vi "בדיקת צריכת זרם של סליל הפיקוד 4.vi"(7 "resultUserPrompt":bool, 8 "error":errorcluster, 11 "Path for Log":path) -> (0 "error out":errorcluster, 2 "צריכת זרם בסליל בטווח כן/לא":bool, 3 "צריכת זרם בסליל":dbl format="%.4f")   [LabVIEW 2015]
uses:
  <vilib>/DAQmx/write.llb/DAQmx Write (Digital Bool 1Line 1Point).vi
  <vilib>/DAQmx/create/channels.llb/DAQmx Create Channel (DO-Digital Output).vi
  <vilib>/DAQmx/miscellaneous.llb/DAQmx Fill In Error Info.vi
panel:
  # "Right-Click to\nexplain error"
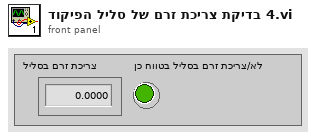
[diagram p1: front panel]
types:
  T1 = enum32{"Invalid", "Standard", "Closed", "Hidden", "Minimized", "Maximized"}
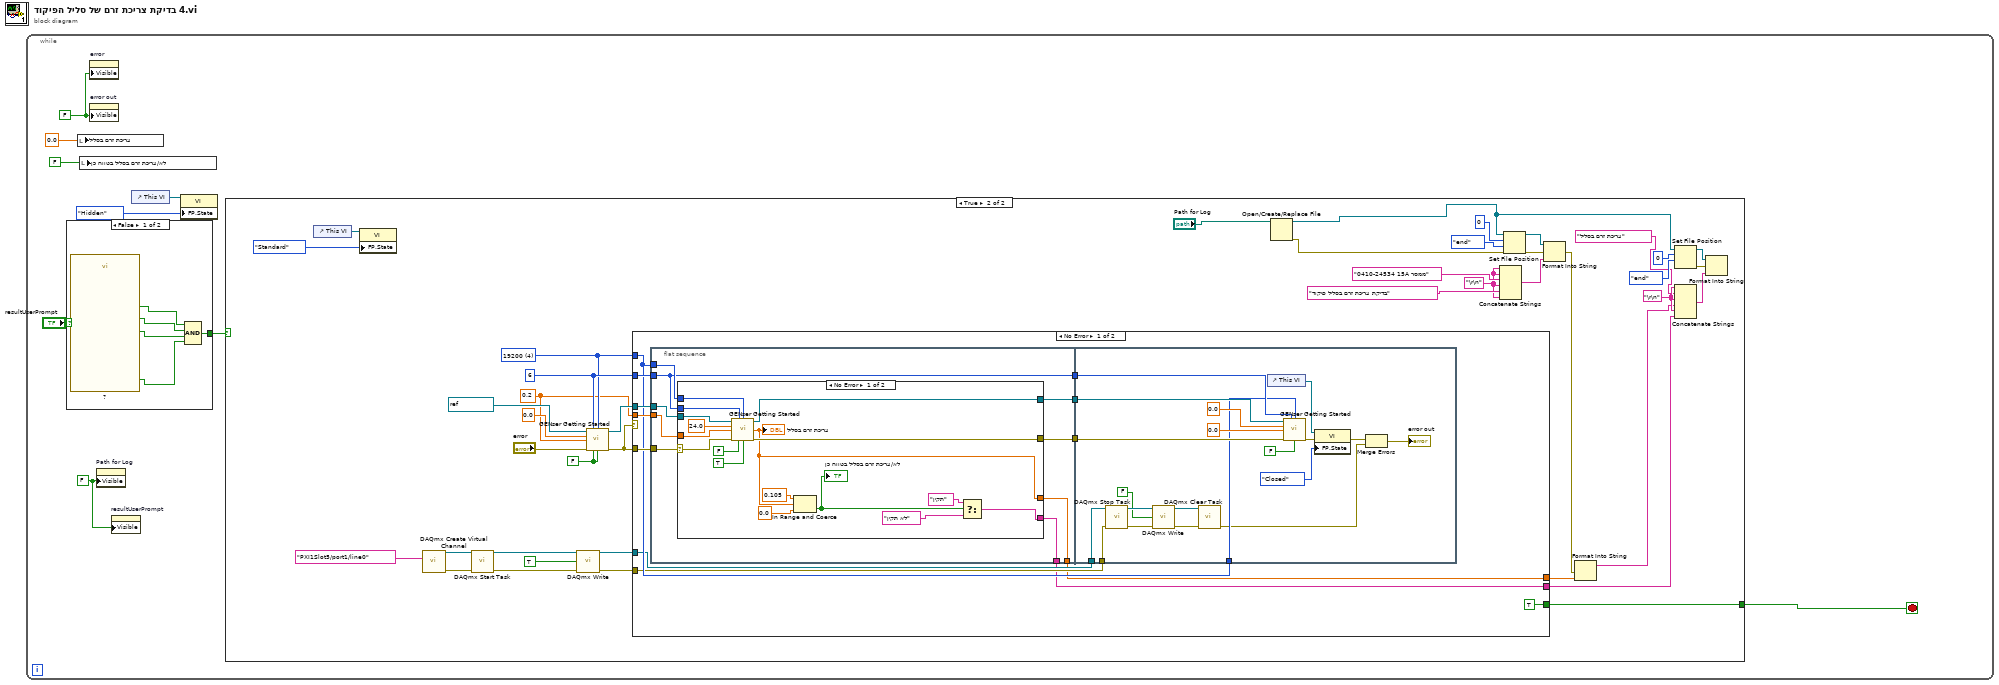
[diagram p0: block diagram]
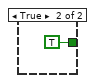
[diagram p2: hidden frame]
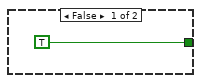
[diagram p3: hidden frame]
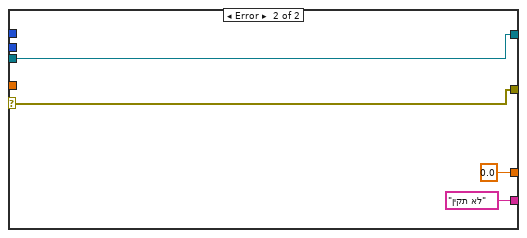
[diagram p4: hidden frame]
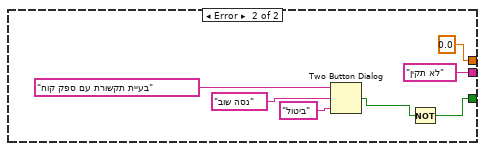
[diagram p5: hidden frame]
diagram:
  n1 = while {
    stop <- w1 stop-if-true
    w2 = FALSE ("Visible")
    w6 = FALSE ("Visible")
    n2 = case shown="False" "resultUserPrompt" {
      tunnel: [w14 TRUE] -> w9
      frame False {
        n3 = call "?"() -> ("הדקי הרב מודד"=w10:bool, "(מגע שלילי (מעטפת"=w11:bool, "A מגע חיובי"=w12:bool, "OK"=w13:bool)  [unwired: 15 in, 1 out]
        n4 = Compound Arithmetic op=AND(w13, w12, w11, w10) -> (w14:bool)
      }
      frame True {
      }
    }
    n5 = local write "צריכת זרם בסליל"(0.0 ("Output Current")) -> ()
    n6 = local write "צריכת זרם בסליל בטווח כן/לא"(FALSE ("In Range?")) -> ()
    n7 = property on="error" class="Clust (strict)"("Visible"=w6) -> ()  [unwired: 2 in, 2 out]
    n8 = property on="error out" class="Clust (strict)"("Visible"=w6) -> ()  [unwired: 2 in, 2 out]
    n9 = property on="Path for Log" class="Path"("Visible"=w2) -> ()  [unwired: 2 in, 2 out]
    n10 = property on="resultUserPrompt" class="Bool (strict)"("Visible"=w2) -> ()  [unwired: 2 in, 2 out]
    n11 = control-ref of="This VI"() -> (w5:refnum<vi>)
    n12 = property class="VI"(reference=w5, "FP.State"=T1."Hidden" ("Front Panel Window:State")) -> ()  [unwired: 1 in, 2 out]
    n13 = case shown="True" w9 {
      tunnel: [TRUE ("T button?") w50] -> w1
      frame False {
      }
      frame True {
        w23 = "\r\n"
        w32 = "\r\n"
        w49 = FALSE ("Output On (T)")
        w54 = u16 4 items=["1200", "2400", "4800", "9600", "19200"] ("BAUD")
        w55 = i16 6 ("GEN Addr")
        w51 = 0.2 ("Current Limit")
        n14 = control-ref of="This VI"() -> (w48:refnum<vi>)
        n15 = property class="VI"(reference=w48, "FP.State"=T1."Standard" ("Front Panel Window:State")) -> ()  [unwired: 1 in, 2 out]
        n16 = call-poly <vilib>:"DAQmx Create Virtual Channel.vi"("lines"=tag "PXI1Slot5/port1/line0") -> ("task out"=w45:refnum<k21>, "error out"=w46:errorcluster)  [unwired: 13 in]
        n17 = call <vilib>:"DAQmx Start Task.vi"("task/channels in"=w45, "error in"=w46) -> ("task out"=w43:refnum<k21>, "error out"=w42:errorcluster)  [unwired: 12 in]
        n18 = call-poly <vilib>:"DAQmx Write.vi"("task/channels in"=w43, "data"=TRUE, "error in"=w42) -> ("task out"=w40:refnum<k21>, "error out"=w39:errorcluster)  [unwired: 10 in, 1 out]
        n19 = call "GENser Getting Started.vi"("VISA"=refnum<visa-resource-name> "COM6", "GEN Addr"=w55, "BAUD"=w54, "Voltage Limit"=0.0, "Current Limit"=w51, "error"="error", "Reset (T)"=w49, "Output On (T)"=w49) -> ("VISA out"=w56:refnum<visa-resource-name>, "error out"=w57:errorcluster)  [unwired: 4 in, 2 out]
        n20 = case shown="No Error" w57 {
          tunnel: w57 -> [w66 _]
          tunnel: w56 -> [w68 _]
          tunnel: w55 -> [w69 _]
          tunnel: w54 -> [w63 _]
          tunnel: w51 -> [w67 _]
          tunnel: [TRUE w122] -> w50
          tunnel: w40 -> [w62 _]
          tunnel: w39 -> [w61 _]
          tunnel: [w60 0.0 ("Output Current")] -> w29
          tunnel: [w59 "לא תקין"] -> w21
          frame No Error {
            n21 = flat-sequence {
              tunnel: [w80] -> w70
              tunnel: w63 -> [w79]
              tunnel: w69 -> [w75]
              tunnel: w68 -> [w78]
              tunnel: w67 -> [w77]
              tunnel: w66 -> [w74]
              tunnel: [w76] -> w65
              tunnel: [w75] -> w64
              tunnel: [w73] -> w60
              tunnel: [w72] -> w59
              tunnel: w70 -> [w118]
              tunnel: w65 -> [w117]
              tunnel: w64 -> [w116]
              tunnel: w63 -> [w115]
              tunnel: w62 -> [w103]
              tunnel: w61 -> [w102]
              frame #0 {
                n22 = case shown="No Error" w74 {
                  selector: w74 -> [w86 w100]
                  tunnel: [w92 w100] -> w80
                  tunnel: w79 -> [w91 _]
                  tunnel: w75 -> [w90 _]
                  tunnel: w78 -> [w89 w101]
                  tunnel: w77 -> [w88 _]
                  tunnel: [w87 w101] -> w76
                  tunnel: [w85 0.0 ("Output Current")] -> w73
                  tunnel: [w81 "לא תקין"] -> w72
                  frame No Error {
                    n23 = call "GENser Getting Started.vi"("VISA"=w89, "GEN Addr"=w90, "BAUD"=w91, "Voltage Limit"=24.0, "Current Limit"=w88, "error"=w86, "Reset (T)"=FALSE, "Output On (T)"=TRUE) -> ("VISA out"=w87:refnum<visa-resource-name>, "Output Current"=w85:dbl, "error out"=w92:errorcluster)  [unwired: 4 in, 1 out]
                    "צריכת זרם בסליל" <- w85
                    n24 = In Range and Coerce(upper limit=0.105, x=w85, lower limit=0.0) -> (In Range?=w82:bool)  [unwired: 1 out]
                    "צריכת זרם בסליל בטווח כן/לא" <- w82
                    n25 = Select(t="תקין", s=w82, f="לא תקין") -> (s? t:f=w81:string)
                  }
                  frame Error {
                  }
                }
              }
              frame #1 {
                n26 = call <vilib>:"DAQmx Stop Task.vi"("task/channels in"=w103, "error in"=w102) -> ("task out"=w111:refnum<k21>, "error out"=w110:errorcluster)  [unwired: 12 in]
                n27 = call-poly <vilib>:"DAQmx Write.vi"("task/channels in"=w111, "data"=FALSE, "error in"=w110) -> ("task out"=w109:refnum<k21>, "error out"=w108:errorcluster)  [unwired: 10 in, 1 out]
                n28 = call <vilib>:"DAQmx Clear Task.vi"("task in"=w109, "error in"=w108) -> ("error out"=w105:errorcluster)  [unwired: 13 in]
                n29 = control-ref of="This VI"() -> (w114:refnum<vi>)
                n30 = call "GENser Getting Started.vi"("VISA"=w117, "GEN Addr"=w116, "BAUD"=w115, "Voltage Limit"=0.0, "Current Limit"=0.0, "error"=w118, "Output On (T)"=FALSE) -> ("error out"=w112:errorcluster)  [unwired: 5 in, 3 out]
                n31 = property class="VI"(reference=w114, error in=w112, "FP.State"=T1."Closed" ("Front Panel Window:State")) -> (error out=w106:errorcluster)  [unwired: 1 out]
                n32 = Merge Errors(w106, w105) -> (→"error out":errorcluster)
              }
            }
          }
          frame Error {
            n33 = Two Button Dialog(message="בעיית תקשורת עם ספק קוח", 1:"ביטול" ("F button name (\"Cancel\")"), 2:"נסה שוב" ("T button name (\"OK\")")) -> (T button?=w123:bool)
            n34 = Not(x=w123) -> (.not. x?=w122:bool)
          }
        }
        n35 = Open/Create/Replace File(file path (use dialog)="Path for Log") -> (refnum out=w17:refnum<file>, error out=w18:errorcluster)  [unwired: 5 in, 1 out]
        n36 = Concatenate Strings(w32, w32, "0410-24534 15A ממסר", w32, "בדיקת צריכת זרם בסליל פיקוד", w32) -> (w36:string)
        n37 = Set File Position(offset (in bytes) (0)=i64 0, refnum=w17, from (0:start)=enum16{"start", "end", "current"}."end", error in=w18) -> (refnum out=w33:refnum<file>, error out=w31:errorcluster)
        n38 = Format Into String(initial string=w33, error in=w31, w36) -> (error out=w30:errorcluster)  [unwired: 1 in, 1 out]
        n39 = Format Into String(error in=w30, w29) -> (resulting string=w20:string)  [unwired: 2 in, 1 out]
        n40 = Set File Position(offset (in bytes) (0)=i64 0, refnum=w17, from (0:start)=enum16{"start", "end", "current"}."end") -> (refnum out=w26:refnum<file>, error out=w27:errorcluster)  [unwired: 1 in]
        n41 = Concatenate Strings(w23, "צריכת זרם בסליל", w23, w20, w23, w21) -> (w28:string)
        n42 = Format Into String(initial string=w26, error in=w27, w28) -> ()  [unwired: 1 in, 2 out]
      }
    }
  }
